vi "Load SubPanel.vi"(8 "error in (no error)":errorcluster, 10 "Clone Name":string, 11 "RootActor in":refnum<class "RootActor.lvclass">) -> (0 "error out":errorcluster, 3 "RootActor out":refnum<class "RootActor.lvclass">)   [LabVIEW 2020, in "RootActor.lvlib" / "RootActor.lvclass"]
uses:
  RootActor.lvclass
  RootActor.lvclass/RootActor.ctl
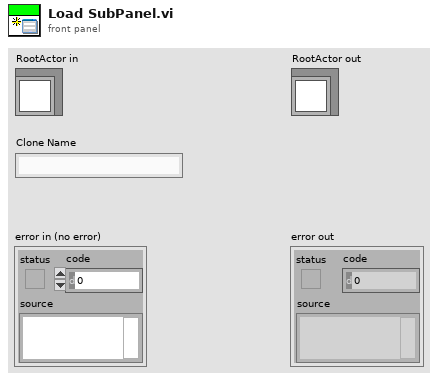
[diagram p1: front panel]
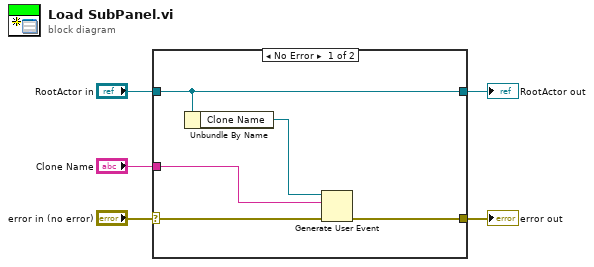
[diagram p0: block diagram]
diagram:
  n1 = case shown="No Error" "error in (no error)" {
    selector: "error in (no error)" -> [w10 w12]
    tunnel: [w9 w12] -> w4
    tunnel: [w8 w11] -> w2
    tunnel: "RootActor in" -> [w8 w11]
    tunnel: "Clone Name" -> [w6 _]
    frame No Error {
      n2 = Unbundle By Name(w8) -> ("Clone Name"=w7:refnum<user-event>)
      n3 = Generate User Event(user event=w7, event data cluster=w6, error in=w10) -> (error out=w9:errorcluster)  [unwired: 1 in, 1 out]
    }
    frame Error {
    }
  }
  "error out" <- w4
  "RootActor out" <- w2
